vi "Record Floor X.vi"(9 "Record":bool, 10 "EncoderDevRef":T1={"DevStatus"={"status"=FALSE, "code"=0, "source"=""}, "EncoderIndex"=enum."Enc 0", "CounterIndex"=enum."Invalid", "DistancePerCount"=1.0, "Decoding Type"=enum."4x"}) -> (1 "New Recording":bool, 2 "Encoder Recording Data":cluster{dbl, u32}[](array[cluster]))   [LabVIEW 2017]
uses:
  <vilib>/Rock Robotics/WPI/Encoder/WPI_EncoderDevRef.ctl
  <vilib>/Rock Robotics/SystemInterfaces/Encoder/FPGA_EncoderIdx.ctl
  <vilib>/Rock Robotics/SystemInterfaces/Counter/FPGA_CounterCtrSystemIndex.ctl
  <vilib>/Rock Robotics/WPI/Encoder/WPI_EncoderType.ctl
panel:
  out "Elapsed Time":u32=1582
  out "Recording Graph":cluster{"Distance":dbl, u32}[](graph)=[{"Distance"=21.0, 0}, {"Distance"=0.0, 20}, {"Distance"=0.0, 40}, {"Distance"=0.0, 61}, {"Distance"=0.0, 81}, {"Distance"=0.0, 102}, {"Distance"=0.0, 122}, {"Distance"=0.0, 143}, {"Distance"=0.0, 163}, {"Distance"=0.0, 184}, {"Distance"=0.0, 204}, {"Distance"=0.0, 224}, {"Distance"=0.0, 245}, {"Distance"=0.0, 265}, {"Distance"=0.0, 285}, {"Distance"=0.0, 305}, {"Distance"=0.0, 325}, {"Distance"=0.0, 346}, {"Distance"=0.0, 366}, {"Distance"=0.0, 387}, {"Distance"=0.0, 407}, {"Distance"=0.0, 428}, {"Distance"=0.0, 448}, {"Distance"=0.0, 468}, {"Distance"=0.0, 488}, {"Distance"=0.0, 508}, {"Distance"=0.0, 529}, {"Distance"=0.0, 549}, {"Distance"=0.0, 569}, {"Distance"=0.0, 589}, {"Distance"=0.0, 609}, {"Distance"=0.0, 629}, {"Distance"=0.0, 649}, {"Distance"=0.0, 669}, {"Distance"=0.0, 690}, {"Distance"=0.0, 710}, {"Distance"=0.0, 730}, {"Distance"=0.0, 750}, {"Distance"=0.0, 770}, {"Distance"=0.0, 791}, {"Distance"=0.0, 811}, {"Distance"=0.0, 831}, {"Distance"=0.0, 851}, {"Distance"=0.0, 872}, {"Distance"=0.0, 892}, {"Distance"=0.0, 913}, {"Distance"=0.0, 933}, {"Distance"=0.0, 953}, {"Distance"=0.0, 973}, {"Distance"=0.0, 993}, {"Distance"=0.0, 1013}, {"Distance"=0.0, 1034}, {"Distance"=0.0, 1054}, {"Distance"=0.0, 1074}, {"Distance"=0.0, 1094}, {"Distance"=0.0, 1114}, {"Distance"=0.0, 1134}, {"Distance"=0.0, 1155}, {"Distance"=0.0, 1175}, {"Distance"=0.0, 1196}, {"Distance"=0.0, 1216}, {"Distance"=0.0, 1236}, {"Distance"=0.0, 1256}, {"Distance"=0.0, 1276}, {"Distance"=0.0, 1297}, {"Distance"=0.0, 1317}, {"Distance"=0.0, 1337}, {"Distance"=0.0, 1358}, {"Distance"=0.0, 1378}, {"Distance"=0.0, 1399}, {"Distance"=0.0, 1419}, {"Distance"=0.0, 1439}, {"Distance"=0.0, 1460}, {"Distance"=0.0, 1480}, {"Distance"=0.0, 1500}, {"Distance"=0.0, 1521}, {"Distance"=0.0, 1541}, {"Distance"=0.0, 1562}, {"Distance"=0.0, 1582}]
  out "Encoder Distance":dbl
  # "Record is used to start/stop recording\n-Starting a new recording wipes out the old one"
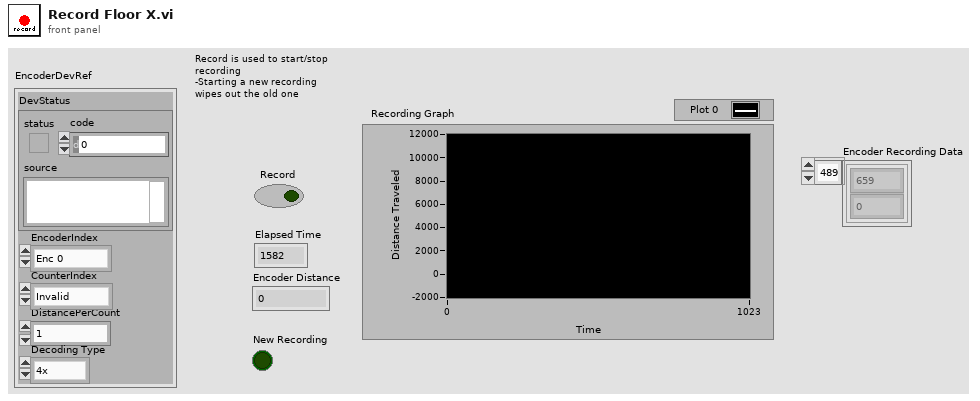
[diagram p1: front panel]
types:
  T1 = typedef "WPI_EncoderDevRef.ctl" = cluster{"DevStatus":errorcluster, "EncoderIndex":T2, "CounterIndex":T3, "DistancePerCount":dbl, "Decoding Type":T4}
  T2 = typedef "FPGA_EncoderIdx.ctl" = enum8{"Enc 0", "Enc 1", "Enc 2", "Enc 3", "Enc 4", "Enc 5", "Enc 6", "Enc 7", "Invalid"}
  T3 = typedef "FPGA_CounterCtrSystemIndex.ctl" = enum8{"Ctr 0", "Ctr 1", "Ctr 2", "Ctr 3", "Ctr 4", "Ctr 5", "Ctr 6", "Ctr 7", "Invalid"}
  T4 = typedef "WPI_EncoderType.ctl" = enum16{"1x", "2x", "4x"}
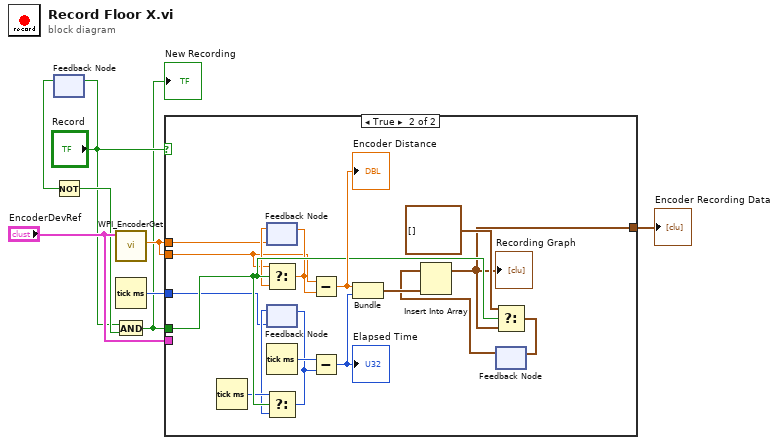
[diagram p0: block diagram]
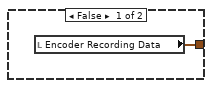
[diagram p2: hidden frame]
diagram:
  n1 = feedback-in #1("Record") -> ()
  n2 = feedback #1() -> (w4:bool)  [unwired: 1 in]
  n3 = Not(x=w4) -> (.not. x?=w3:bool)
  n4 = call <vilib>:"WPI_EncoderGet.vi"("EncoderDevRef"="EncoderDevRef") -> ("Distance"=w5:dbl)  [unwired: 5 in, 5 out]
  n5 = Tick Count (ms)() -> (millisecond timer value=w6:u32)
  n6 = And(x="Record", y=w3) -> (x .and. y?=w1:bool)
  "New Recording" <- w1
  n7 = case shown="True" "Record" {
    tunnel: "EncoderDevRef" -> [_ _]
    tunnel: [w9 w18] -> w7
    tunnel: w1 -> [_ w19]
    tunnel: w6 -> [_ w12]
    tunnel: w5 -> [_ w11]
    tunnel: w5 -> [_ w10]
    frame False {
      n8 = local read "Encoder Recording Data"() -> (w9:cluster{dbl, u32}[])
    }
    frame True {
      n9 = Tick Count (ms)() -> (millisecond timer value=w17:u32)
      n10 = feedback #2(w10) -> (w16:dbl)
      n11 = Select(t=w11, s=w19, f=w16) -> (s? t:f=w13:dbl)
      n12 = feedback-in #2(w13) -> ()
      n13 = feedback #3(w12) -> (w15:u32)
      n14 = Tick Count (ms)() -> (millisecond timer value=w25:u32)
      n15 = Select(t=w17, s=w19, f=w15) -> (s? t:f=w14:u32)
      n16 = feedback-in #3(w14) -> ()
      n17 = Subtract(x=w11, y=w13) -> (x-y=w23:dbl)
      "Encoder Distance" <- w23
      n18 = Subtract(x=w25, y=w14) -> (x-y=w24:u32)
      "Elapsed Time" <- w24
      n19 = Bundle(w23, w24) -> (w26:cluster{dbl, u32})  [unwired: 1 in]
      n20 = feedback #4() -> (w22:cluster{dbl, u32}[])  [unwired: 1 in]
      n21 = Insert Into Array(array=w22, new element=w26) -> (w18:cluster{dbl, u32}[])  [unwired: 1 in]
      "Recording Graph" <- w18
      n22 = Select(t=cluster{dbl, u32}[] [], s=w19, f=w18) -> (s? t:f=w20:cluster{dbl, u32}[])
      n23 = feedback-in #4(w20) -> ()
    }
  }
  "Encoder Recording Data" <- w7
